vi "Stage Forward.vi"(8 "error in (no error)":errorcluster, 11 "Application in":refnum<class "Application.lvclass">) -> (0 "error out":errorcluster, 3 "Application out":refnum<class "Application.lvclass">)   [LabVIEW 2018, in "Application.lvlib" / "Application.lvclass"]
uses:
  Application.lvclass
  Application.lvclass/Application.ctl
  <vilib>/ActorFramework/Message Enqueuer/Message Enqueuer.lvclass/Message Enqueuer.ctl
  <vilib>/ActorFramework/Message Enqueuer/Enqueue.vi
  Hardware/Stage Controller Messages/Move Forward Msg/Move Forward Msg.lvclass
  C:/Program Files/National Instruments/LabVIEW 2018/vi.lib/ActorFramework/Message/Message.lvclass
  <vilib>/ActorFramework/Message Priority Queue/Priority Enqueue.vi
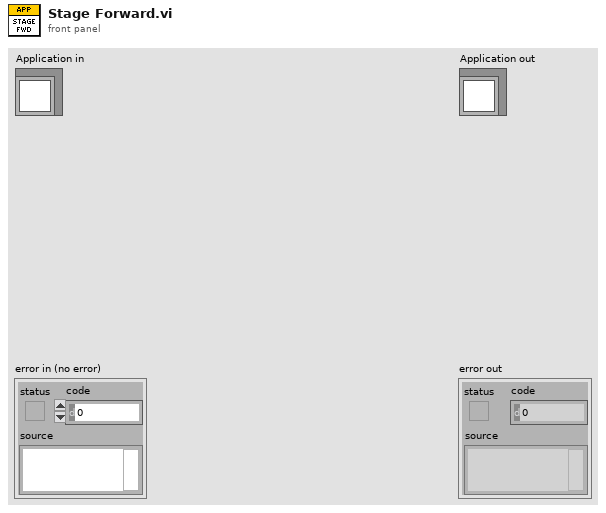
[diagram p1: front panel]
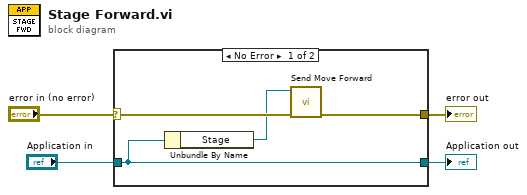
[diagram p0: block diagram]
diagram:
  n1 = case shown="No Error" "error in (no error)" {
    selector: "error in (no error)" -> [w7 w10]
    tunnel: [w6 w10] -> w3
    tunnel: [w8 w9] -> w1
    tunnel: "Application in" -> [w8 w9]
    frame No Error {
      n2 = Unbundle By Name(w8) -> ("Stage"=w5:refnum<class "Message Enqueuer.lvclass">)
      n3 = call "Send Move Forward.vi"("error in (no error)"=w7, "Message Enqueuer"=w5) -> ("error out"=w6:errorcluster)  [unwired: 8 in, 1 out]
    }
    frame Error {
    }
  }
  "error out" <- w3
  "Application out" <- w1
